vi "Create_Turbulence_Statistics.vi"() -> ()   [LabVIEW 2011]
uses:
  <vilib>/Analysis/1siggen.llb/Ramp Pattern by Samples.vi
  <vilib>/Utility/file.llb/Write To Spreadsheet File (string).vi
  <vilib>/Analysis/baseanly.llb/Quick Scale 1D.vi
  <vilib>/Analysis/NI_AALBase.lvlib
panel:
  in  "Meas Plane":enum16{"XY", "YZ", "XZ"}(ring)
  in  "Invert V":bool
  in  "Invert U":bool
  in  "Output Directory":path=path "C:/Experiments10/NACA0015_D"
  out "Current vector filename":string
  out "v4 (m4/s4)":dbl(graph)
  out "v3 (m3/s3)":dbl(graph)
  out "v2 (m2/s2)":dbl(graph)
  out "V (m/s)":dbl(graph)
  out "v (m/s)":dbl(graph)
  out "u4 (m4/s4)":dbl(graph)
  out "u3 (m3/s3)":dbl(graph)
  out "u2 (m2/s2)":dbl(graph)
  out "u (m/s)":dbl(graph)
  out "U (m/s)":dbl(graph)
  in  "New Filename":string
  in  "Insight 3G File Folder":path=path "C:/Experiments10/NACA0015_D"
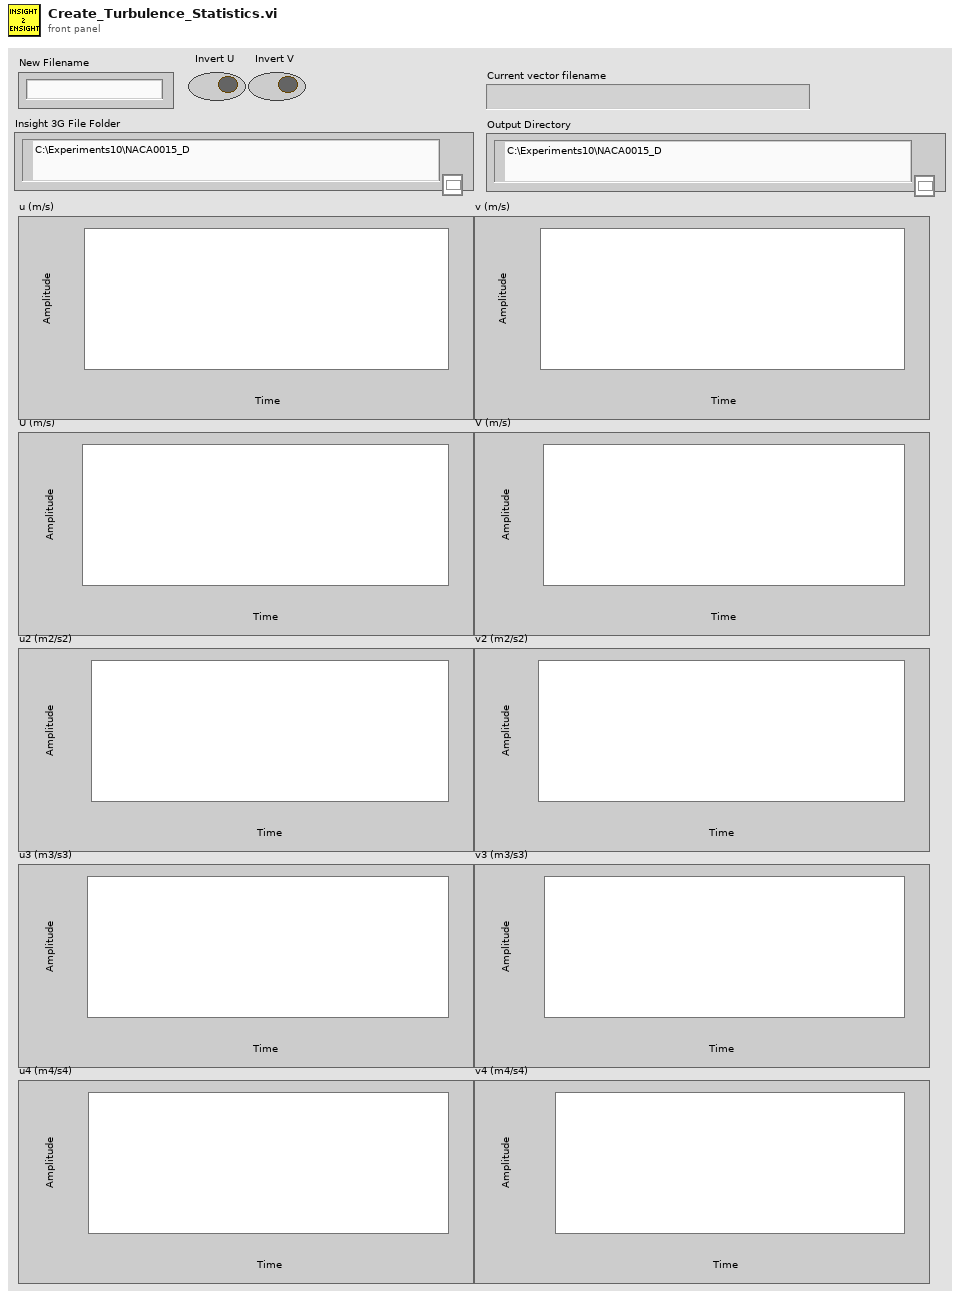
[diagram p1: front panel]
types:
  T1 = cluster{"U m/s":dbl, "u2 m2/s2":dbl, "u3 m3/s3":dbl, "u4 m4/s4":dbl, "TurbU %":dbl, "Skew_u":dbl, "Kurt_u":dbl, "V m/s":dbl, "v2 m2/s2":dbl, "v3 m3/s3":dbl, "v4 m4/s4":dbl, "TurbV %":dbl, "Skew_v":dbl, "Kurt_v":dbl, "u2v2 m4/s4":dbl, "uv3 m4/s4":dbl, "u3v m4/s4":dbl, "uv2 m3/s3":dbl, "u2v m3/s3":dbl, "uv_cc":dbl, "uv":dbl, "TKE J":dbl}
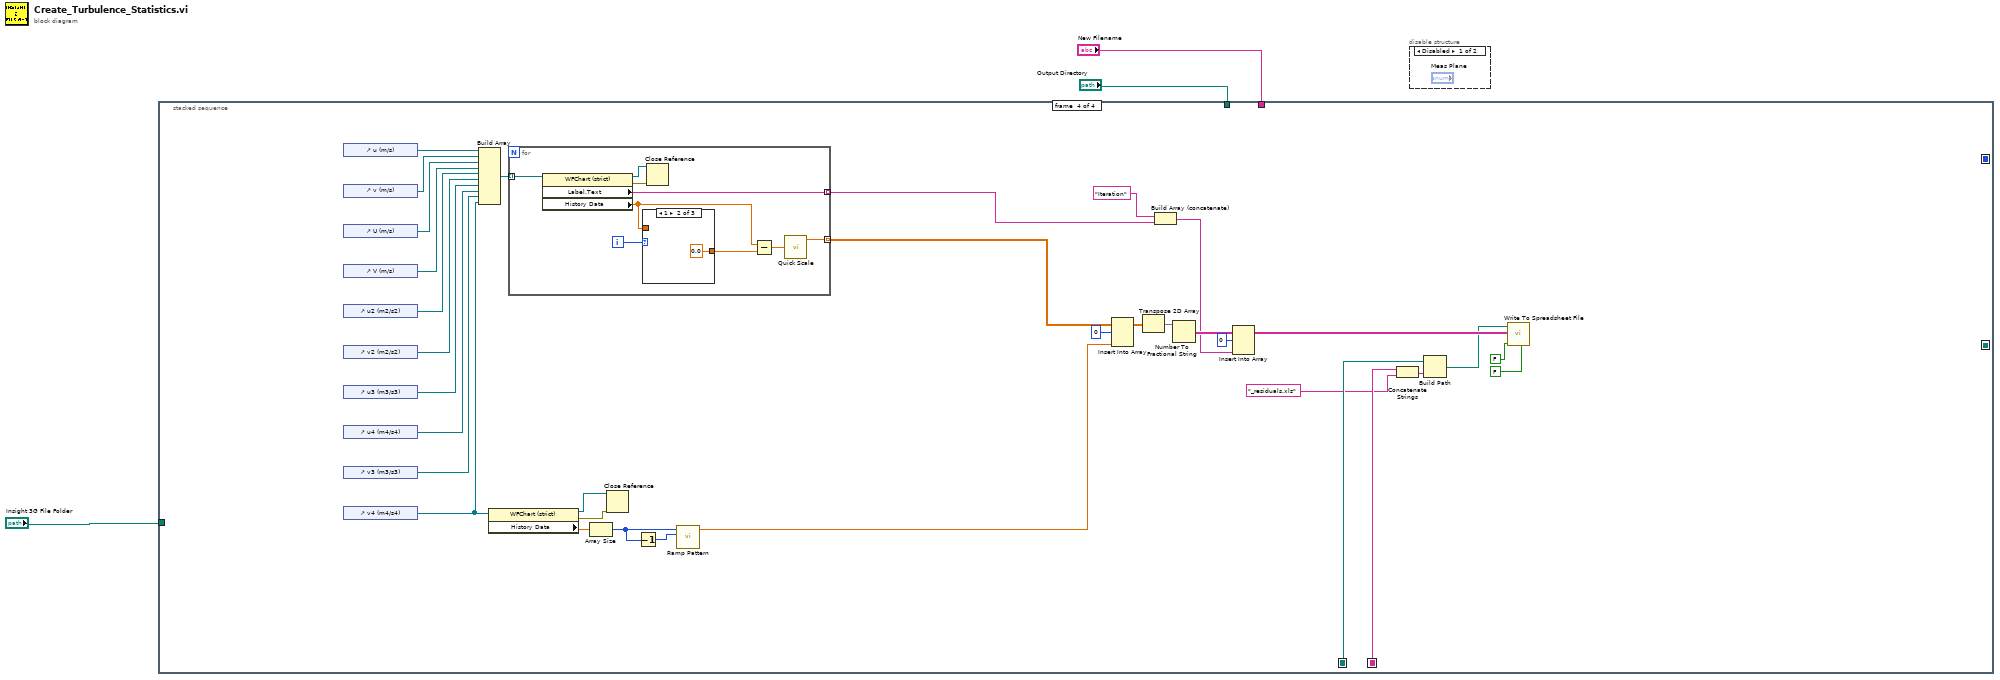
[diagram p0: block diagram]
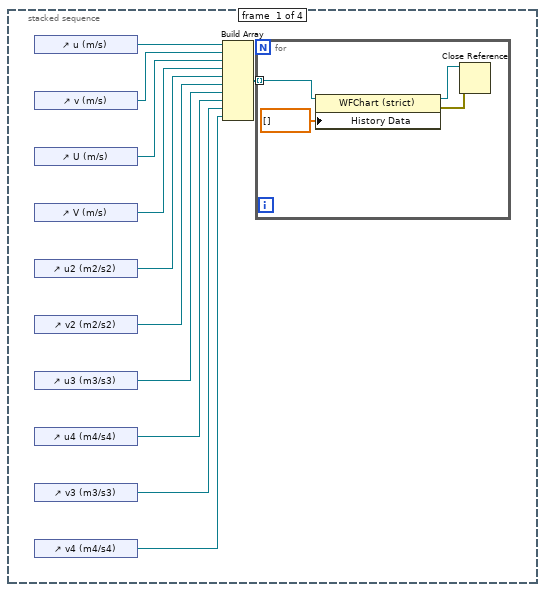
[diagram p3: hidden frame]
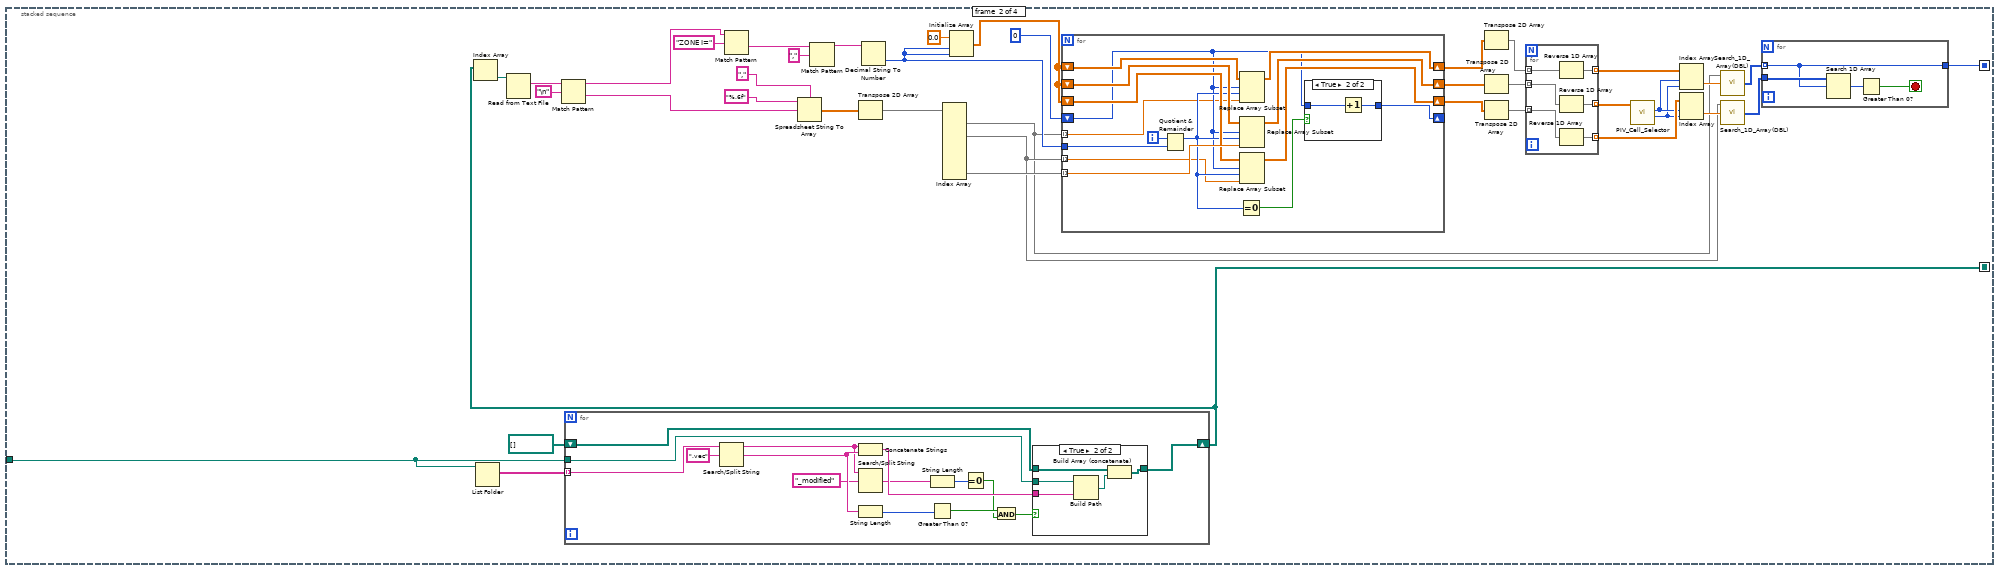
[diagram p4: hidden frame]
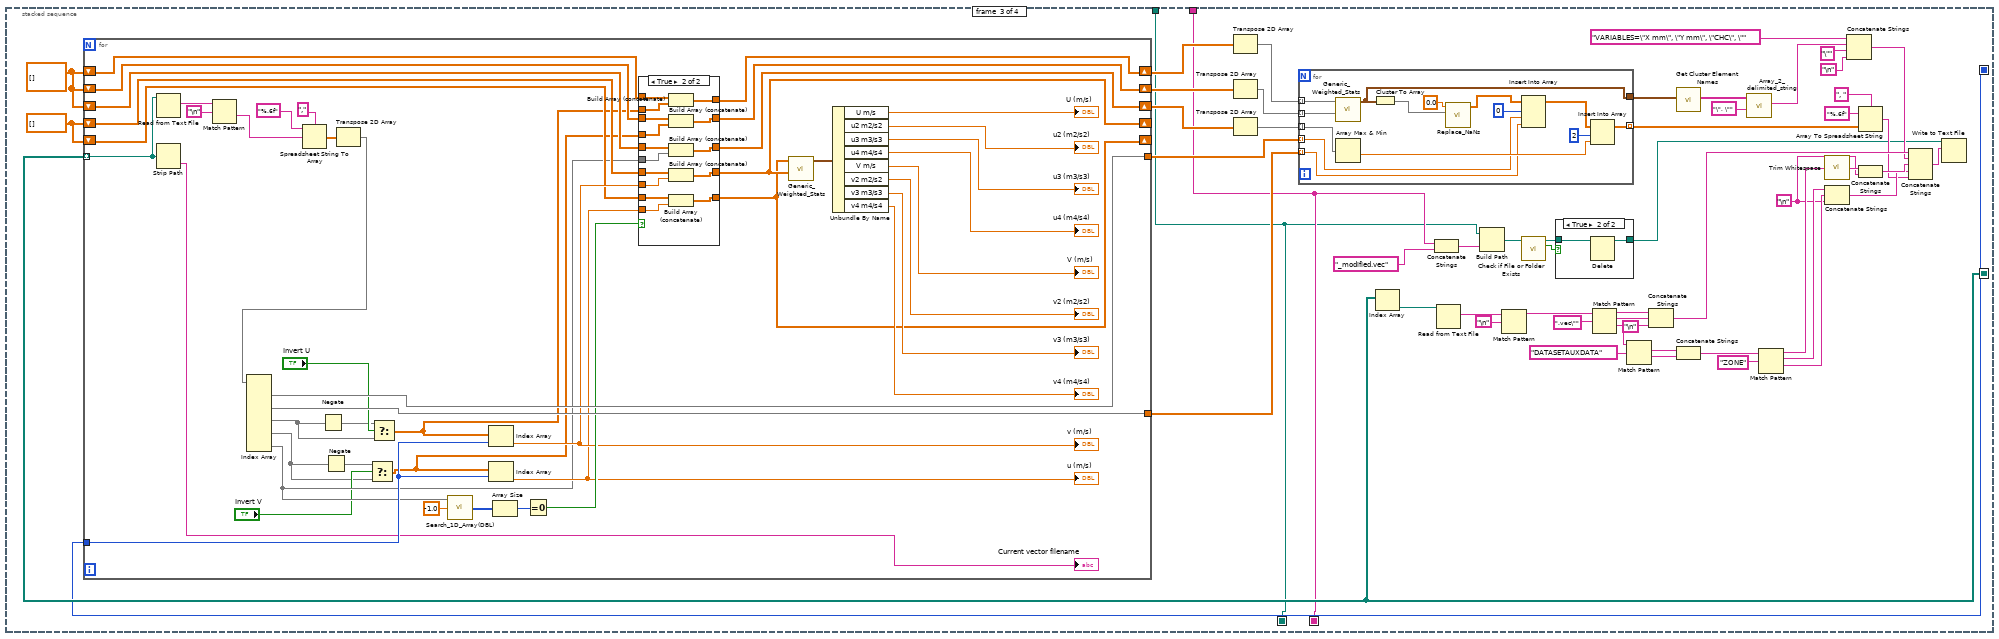
[diagram p7: hidden frame]
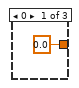
[diagram p10: hidden frame]
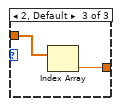
[diagram p11: hidden frame]
diagram:
  n1 = stacked-sequence {
    seq-local: [_ w56 _ _] -> [_ _ w162 _]
    seq-local: [_ w22 _ _] -> [_ _ w161 _]
    seq-local: [_ _ w108 _] -> [_ _ _ w253]
    seq-local: [_ _ w109 _] -> [_ _ _ w249]
    tunnel: "New Filename" -> [_ _ w109 _]
    tunnel: "Output Directory" -> [_ _ w108 _]
    tunnel: "Insight 3G File Folder" -> [_ w19 _ _]
    frame #0 {
      n2 = control-ref of="u (m/s)"() -> (w14:refnum<vi>)
      n3 = control-ref of="v (m/s)"() -> (w13:refnum<vi>)
      n4 = control-ref of="U (m/s)"() -> (w12:refnum<vi>)
      n5 = control-ref of="V (m/s)"() -> (w11:refnum<vi>)
      n6 = control-ref of="u2 (m2/s2)"() -> (w10:refnum<vi>)
      n7 = control-ref of="v2 (m2/s2)"() -> (w9:refnum<vi>)
      n8 = control-ref of="u3 (m3/s3)"() -> (w8:refnum<vi>)
      n9 = control-ref of="u4 (m4/s4)"() -> (w7:refnum<vi>)
      n10 = control-ref of="v3 (m3/s3)"() -> (w6:refnum<vi>)
      n11 = control-ref of="v4 (m4/s4)"() -> (w4:refnum<vi>)
      n12 = Build Array(w14, w13, w12, w11, w10, w9, w8, w7, w6, w4) -> (w5:refnum<vi>[])
      n13 = for {
        tunnel: w5 -> [w18] mode=indexing
        n14 = property class="WFChart (strict)"(reference=w18, "History Data"=dbl[] []) -> (reference out=w16:refnum<vi>, error out=w17:errorcluster)  [unwired: 1 in]
        n15 = Close Reference(reference=w16, error in (no error)=w17) -> ()  [unwired: 1 out]
      }
    }
    frame #1 {
      n16 = List Folder(path=w19) -> (filenames=w57:string[])  [unwired: 3 in, 3 out]
      n17 = for {
        tunnel: w57 -> [w101] mode=indexing
        shift-right: [w94] -> w56
        shift-left: path[] [] -> [w96]
        tunnel: w19 -> [w95]
        n18 = Search/Split String(string=w101, search string/char (-)=".vec") -> (substring before match=w92:string, match + rest of string=w98:string)  [unwired: 1 in, 1 out]
        n19 = Concatenate Strings(w92, w98) -> (w97:string)
        n20 = Search/Split String(string=w92, search string/char (-)="_modified") -> (match + rest of string=w90:string)  [unwired: 1 in, 2 out]
        n21 = String Length(string=w98) -> (length=w99:i32)
        n22 = Greater Than 0?(x=w99) -> (x > 0?=w93:bool)
        n23 = String Length(string=w90) -> (length=w89:i32)
        n24 = Equal To 0?(x=w89) -> (x = 0?=w88:bool)
        n25 = And(x=w93, y=w88) -> (x .and. y?=w87:bool)
        n26 = case shown="True" w87 {
          tunnel: w97 -> [_ w107]
          tunnel: w96 -> [w102 w103]
          tunnel: w95 -> [_ w106]
          tunnel: [w102 w104] -> w94
          frame False {
          }
          frame True {
            n27 = Build Path(base path=w106, name or relative path=w107) -> (appended path=w105:path)
            n28 = Build Array (concatenate)(w103, w105) -> (w104:path[])
          }
        }
      }
      n29 = Index Array(array=w56) -> (element=w55:path)  [unwired: 1 in]
      n30 = Read from Text File(file (use dialog)=w55) -> (text=w48:string)  [unwired: 3 in, 3 out]
      n31 = Match Pattern(string=w48, regular expression="\n") -> (before substring=w47:string, after substring=w51:string)  [unwired: 1 in, 2 out]
      n32 = Match Pattern(string=w47, regular expression="ZONE I=") -> (after substring=w45:string)  [unwired: 1 in, 3 out]
      n33 = Spreadsheet String To Array(delimiter (Tab)=",", format string="%.6f", spreadsheet string=w51) -> (array=w50:dbl[][])  [unwired: 1 in]
      n34 = Match Pattern(string=w45, regular expression=",") -> (before substring=w43:string)  [unwired: 1 in, 3 out]
      n35 = Transpose 2D Array(2D array=w50) -> (transposed array=w53:dbl[][])
      n36 = Decimal String To Number(string=w43) -> (number=w27:i32)  [unwired: 2 in, 1 out]
      n37 = Index Array(array=w53) -> (element #1=w23:dbl[], element #2=w24:dbl[], element #5=w42:dbl[])  [unwired: 10 in, 2 out]
      n38 = Initialize Array(0.0 ("element"), w27, w27) -> (w36:dbl[][])
      n39 = for {
        tunnel: w42 -> [w79] mode=indexing
        tunnel: w27 -> [w82]
        shift-right: [w80] -> w39
        shift-left: w36 -> [w81]
        shift-right: [w78] -> _
        shift-left: 0 -> [w71]
        shift-right: [w76] -> w34
        shift-left: w36 -> [w75]
        shift-right: [w73] -> w35
        shift-left: w36 -> [w74]
        tunnel: w23 -> [w70] mode=indexing
        tunnel: w24 -> [w69] mode=indexing
        i -> [w83]
        n40 = Quotient & Remainder(x=w83, y=w82) -> (x-y*floor(x/y)=w72:i32)  [unwired: 1 out]
        n41 = Equal To 0?(x=w72) -> (x = 0?=w77:bool)
        n42 = Replace Array Subset(array=w74, new element=w70, index (row)=w71, index (col)=w72) -> (w73:dbl[][])
        n43 = Replace Array Subset(array=w81, new element=w79, index (row)=w71, index (col)=w72) -> (w80:dbl[][])
        n44 = Replace Array Subset(array=w75, new element=w69, index (row)=w71, index (col)=w72) -> (w76:dbl[][])
        n45 = case shown="True" w77 {
          tunnel: [w84 w85] -> w78
          tunnel: w71 -> [w84 w86]
          frame False {
          }
          frame True {
            n46 = Increment(x=w86) -> (x+1=w85:i32)
          }
        }
      }
      n47 = Transpose 2D Array(2D array=w35) -> (transposed array=w33:dbl[][])
      n48 = Transpose 2D Array(2D array=w39) -> (transposed array=w38:dbl[][])
      n49 = Transpose 2D Array(2D array=w34) -> (transposed array=w32:dbl[][])
      n50 = for {
        tunnel: w38 -> [w68] mode=indexing
        tunnel: [w67] -> w37 mode=indexing
        tunnel: w33 -> [w66] mode=indexing
        tunnel: w32 -> [w65] mode=indexing
        tunnel: [w64] -> w30 mode=indexing
        tunnel: [w63] -> w31 mode=indexing
        n51 = Reverse 1D Array(array=w66) -> (reversed array=w63:dbl[])
        n52 = Reverse 1D Array(array=w68) -> (reversed array=w67:dbl[])
        n53 = Reverse 1D Array(array=w65) -> (reversed array=w64:dbl[])
      }
      n54 = call "PIV_Cell_Selector.vi"("CHC"=w37) -> ("Y Index"=w20:i32, "X Index"=w21:i32)  [unwired: 9 in]
      n55 = Index Array(array=w31, index (row)=w21, index (col)=w20) -> (element=w29:dbl)
      n56 = Index Array(array=w30, index (row)=w21, index (col)=w20) -> (element=w28:dbl)
      n57 = call "Search_1D_Array(DBL).vi"("Array"=w23, "Element Data"=w29) -> ("Indicies of Elements"=w26:i32[])  [unwired: 7 in]
      n58 = call "Search_1D_Array(DBL).vi"("Array"=w24, "Element Data"=w28) -> ("Indicies of Elements"=w25:i32[])  [unwired: 7 in]
      n59 = for {
        tunnel: w26 -> [w59] mode=indexing
        tunnel: w25 -> [w62]
        tunnel: [w59] -> w22
        stop <- w60 stop-if-true
        n60 = Search 1D Array(1D array=w62, element=w59) -> (index of element=w61:i32)  [unwired: 1 in]
        n61 = Greater Than 0?(x=w61) -> (x > 0?=w60:bool)
      }
    }
    frame #2 {
      w114 = dbl[][] []
      w115 = dbl[] []
      w134 = "\n"
      n62 = for {
        tunnel: w162 -> [w204] mode=indexing
        tunnel: [w218] -> w123
        tunnel: [w217] -> w122
        tunnel: w161 -> [w216]
        shift-right: [w194] -> _
        shift-left: w115 -> [w195]
        shift-right: [w197] -> _
        shift-left: w115 -> [w198]
        shift-right: [w189] -> w112
        shift-left: w114 -> [w191]
        shift-right: [w188] -> w111
        shift-left: w114 -> [w190]
        shift-right: [w193] -> w113
        shift-left: w114 -> [w200]
        n63 = Read from Text File(file (use dialog)=w204) -> (text=w221:string)  [unwired: 3 in, 3 out]
        n64 = Strip Path(path=w204) -> (name=→"Current vector filename":string)  [unwired: 1 out]
        n65 = Match Pattern(string=w221, regular expression="\n") -> (after substring=w220:string)  [unwired: 1 in, 3 out]
        n66 = Spreadsheet String To Array(delimiter (Tab)=",", format string="%.6f", spreadsheet string=w220) -> (array=w219:dbl[][])  [unwired: 1 in]
        n67 = Transpose 2D Array(2D array=w219) -> (transposed array=w223:dbl[][])
        n68 = Index Array(array=w223) -> (element #1=w218:dbl[], element #2=w217:dbl[], element #3=w185:dbl[], element #4=w181:dbl[], element #5=w192:dbl[])  [unwired: 10 in]
        n69 = Negate(x=w185) -> (-x=w184:dbl[])
        n70 = Negate(x=w181) -> (-x=w180:dbl[])
        n71 = Select(t=w180, s="Invert V", f=w181) -> (s? t:f=w183:dbl[])
        n72 = Select(t=w184, s="Invert U", f=w185) -> (s? t:f=w186:dbl[])
        n73 = call "Search_1D_Array(DBL).vi"("Array"=w192, "Element Data"=-1.0) -> ("Indicies of Elements"=w205:i32[])  [unwired: 7 in]
        n74 = Index Array(array=w186, index=w216) -> (element=w199:dbl)
        "v (m/s)" <- w199
        n75 = Index Array(array=w183, index=w216) -> (element=w196:dbl)
        "u (m/s)" <- w196
        n76 = Array Size(array=w205) -> (size(s)=w202:i32)
        n77 = Equal To 0?(x=w202) -> (x = 0?=w201:bool)
        n78 = case shown="True" w201 {
          tunnel: w200 -> [w228 w238]
          tunnel: w199 -> [_ w245]
          tunnel: w198 -> [w229 w244]
          tunnel: [w229 w243] -> w197
          tunnel: w196 -> [_ w242]
          tunnel: w195 -> [w230 w241]
          tunnel: [w230 w240] -> w194
          tunnel: w186 -> [_ w239]
          tunnel: [w228 w237] -> w193
          tunnel: w183 -> [_ w236]
          tunnel: w192 -> [_ w235]
          tunnel: w191 -> [w227 w234]
          tunnel: w190 -> [w226 w233]
          tunnel: [w227 w232] -> w189
          tunnel: [w226 w231] -> w188
          frame False {
          }
          frame True {
            n79 = Build Array (concatenate)(w238, w239) -> (w237:dbl[][])
            n80 = Build Array (concatenate)(w234, w236) -> (w232:dbl[][])
            n81 = Build Array (concatenate)(w233, w235) -> (w231:dbl[][])
            n82 = Build Array (concatenate)(w244, w245) -> (w243:dbl[])
            n83 = Build Array (concatenate)(w241, w242) -> (w240:dbl[])
          }
        }
        n84 = call "Generic_Weighted_Stats.vi"("v"=w197, "u"=w194) -> ("Turbulence Statistics"=w215:T1)  [unwired: 9 in]
        n85 = Unbundle By Name(w215) -> ("U m/s"=→"U (m/s)":dbl, "u2 m2/s2"=→"u2 (m2/s2)":dbl, "u3 m3/s3"=→"u3 (m3/s3)":dbl, "u4 m4/s4"=→"u4 (m4/s4)":dbl, "V m/s"=→"V (m/s)":dbl, "v2 m2/s2"=→"v2 (m2/s2)":dbl, "v3 m3/s3"=→"v3 (m3/s3)":dbl, "v4 m4/s4"=→"v4 (m4/s4)":dbl)
      }
      n86 = Transpose 2D Array(2D array=w113) -> (transposed array=w160:dbl[][])
      n87 = Transpose 2D Array(2D array=w112) -> (transposed array=w159:dbl[][])
      n88 = Transpose 2D Array(2D array=w111) -> (transposed array=w124:dbl[][])
      n89 = for {
        tunnel: w160 -> [w179] mode=indexing
        tunnel: w159 -> [w178] mode=indexing
        tunnel: [w174] -> w128 mode=indexing
        tunnel: w123 -> [w172] mode=indexing
        tunnel: w122 -> [w173] mode=indexing
        tunnel: w124 -> [w176] mode=indexing
        tunnel: [w166] -> w117
        n90 = call "Generic_Weighted_Stats.vi"("v"=w178, "u"=w179) -> ("Turbulence Statistics"=w166:T1)  [unwired: 9 in]
        n91 = Array Max & Min(array=w176) -> (min value=w175:dbl)  [unwired: 3 out]
        n92 = Cluster To Array(cluster=w166) -> (array=w169:dbl[])
        n93 = call "Replace_NaNs.vi"("Array"=w169, "Replacement"=0.0 ("t")) -> ("Array Out"=w168:dbl[])  [unwired: 9 in]
        n94 = Insert Into Array(array=w168, index=0, new element #1=w172, new element #2=w173) -> (w170:dbl[])
        n95 = Insert Into Array(array=w170, index=2, new element=w175) -> (w174:dbl[])
      }
      n96 = Index Array(array=w162) -> (element=w154:path)  [unwired: 1 in]
      n97 = Concatenate Strings(w109, "_modified.vec" ("string")) -> (w110:string)
      n98 = Read from Text File(file (use dialog)=w154) -> (text=w157:string)  [unwired: 3 in, 3 out]
      n99 = Build Path(base path=w108, name or relative path=w110) -> (appended path=w133:path)
      n100 = Match Pattern(string=w157, regular expression="\n") -> (before substring=w156:string)  [unwired: 1 in, 3 out]
      n101 = call <vilib>:"Check if File or Folder Exists.vi"("path"=w133) -> ("file or folder exists?"=w120:bool, "dup path"=w119:path)  [unwired: 8 in, 1 out]
      n102 = case shown="True" w120 {
        tunnel: w119 -> [w163 w165]
        tunnel: [w163 w164] -> w118
        frame False {
        }
        frame True {
          n103 = Delete(path (use dialog)=w165) -> (deleted path=w164:path)  [unwired: 4 in, 2 out]
        }
      }
      n104 = Match Pattern(string=w156, regular expression=".vec\"") -> (before substring=w151:string, match substring=w150:string, after substring=w148:string)  [unwired: 1 in, 1 out]
      n105 = Match Pattern(string=w148, regular expression="DATASETAUXDATA") -> (match substring=w146:string, after substring=w145:string)  [unwired: 1 in, 2 out]
      n106 = Concatenate Strings(w151, w150, "\n") -> (w138:string)
      n107 = call "Get Cluster Element Names.vi"("Cluster"=w117) -> ("Element Names"=w116:string[])  [unwired: 9 in, 1 out]
      n108 = Concatenate Strings(w146, w145) -> (w144:string)
      n109 = call "Array_2_delimited_string.vi"("delimiter (Tab)"="\", \"", "Array of Strings"=w116) -> ("delimited string"=w131:string)  [unwired: 9 in]
      n110 = Match Pattern(string=w144, regular expression="ZONE") -> (before substring=w142:string, match substring=w140:string, after substring=w139:string)  [unwired: 1 in, 1 out]
      n111 = call <vilib>:"Trim Whitespace.vi"("string"=w142) -> ("trimmed string"=w141:string)  [unwired: 1 in]
      n112 = Concatenate Strings(w140, w139, w134) -> (w135:string)
      n113 = Concatenate Strings("VARIABLES=\"X mm\", \"Y mm\", \"CHC\", \"" ("string"), w131, "\"" ("string"), "\n") -> (w137:string)
      n114 = Array To Spreadsheet String(delimiter (Tab)=", ", array=w128, 3:"%.6f" ("format string")) -> (spreadsheet string=w125:string)
      n115 = Concatenate Strings(w141, w134) -> (w136:string)
      n116 = Concatenate Strings(w138, w137, w136, w135, w125) -> (w121:string)
      n117 = Write to Text File(file (use dialog)=w118, text=w121) -> ()  [unwired: 2 in, 3 out]
    }
    frame #3 {
      n118 = control-ref of="u (m/s)"() -> (w279:refnum<vi>)
      n119 = control-ref of="v (m/s)"() -> (w278:refnum<vi>)
      n120 = control-ref of="U (m/s)"() -> (w277:refnum<vi>)
      n121 = control-ref of="V (m/s)"() -> (w276:refnum<vi>)
      n122 = control-ref of="u2 (m2/s2)"() -> (w275:refnum<vi>)
      n123 = control-ref of="v2 (m2/s2)"() -> (w274:refnum<vi>)
      n124 = control-ref of="u3 (m3/s3)"() -> (w273:refnum<vi>)
      n125 = control-ref of="u4 (m4/s4)"() -> (w272:refnum<vi>)
      n126 = control-ref of="v3 (m3/s3)"() -> (w271:refnum<vi>)
      n127 = control-ref of="v4 (m4/s4)"() -> (w269:refnum<vi>)
      n128 = Build Array(w279, w278, w277, w276, w275, w274, w273, w272, w271, w269) -> (w270:refnum<vi>[])
      n129 = property class="WFChart (strict)"(reference=w269) -> (reference out=w267:refnum<vi>, error out=w266:errorcluster, "History Data"=w268:dbl[])  [unwired: 1 in]
      n130 = for {
        tunnel: w270 -> [w288] mode=indexing
        tunnel: [w281] -> w264 mode=indexing
        tunnel: [w287] -> w260 mode=indexing
        i -> [w280]
        n131 = property class="WFChart (strict)"(reference=w288) -> (reference out=w285:refnum<vi>, error out=w286:errorcluster, "Label.Text"=w287:string, "History Data"=w284:dbl[])  [unwired: 1 in]
        n132 = case shown="1" w280 {
          tunnel: w284 -> [_ _ w292]
          tunnel: [0.0 0.0 w291] -> w283
          frame 0 {
          }
          frame 1 {
          }
          frame 2, Default {
            n133 = Index Array(array=w292) -> (element=w291:dbl)  [unwired: 1 in]
          }
        }
        n134 = Close Reference(reference=w285, error in (no error)=w286) -> ()  [unwired: 1 out]
        n135 = Subtract(x=w284, y=w283) -> (x-y=w282:dbl[])
        n136 = call-poly <vilib>:"Quick Scale.vi"("X"=w282) -> ("Y[i]=X[i]/Max|X|"=w281:dbl[])  [unwired: 2 out]
      }
      n137 = Array Size(array=w268) -> (size(s)=w265:i32)
      n138 = Close Reference(reference=w267, error in (no error)=w266) -> ()  [unwired: 1 out]
      n139 = Decrement(x=w265) -> (x-1=w246:i32)
      n140 = call-poly <vilib>:"Ramp Pattern.vi"("end"=w246, "samples"=w265) -> ("Ramp Pattern"=w263:dbl[])  [unwired: 8 in, 1 out]
      n141 = Insert Into Array(array=w264, index (row)=0, new element=w263) -> (w261:dbl[][])  [unwired: 1 in]
      n142 = Transpose 2D Array(2D array=w261) -> (transposed array=w258:dbl[][])
      n143 = Build Array (concatenate)("Iteration", w260) -> (w256:string[])
      n144 = Number To Fractional String(number=w258) -> (F-format string=w257:string[][])  [unwired: 3 in]
      n145 = Insert Into Array(array=w257, index (row)=0, new element=w256) -> (w254:string[][])  [unwired: 1 in]
      n146 = Concatenate Strings(w249, "_residuals.xls" ("string")) -> (w248:string)
      n147 = Build Path(base path=w253, name or relative path=w248) -> (appended path=w252:path)
      n148 = call-poly <vilib>:"Write To Spreadsheet File.vi"("transpose? (no:F)"=FALSE, "append to file? (new file:F)"=FALSE, "2D data"=w254, "file path (dialog if empty)"=w252) -> ()  [unwired: 4 in, 1 out]
    }
  }
  n149 = disable-structure shown="Disabled" {
    frame Disabled {
    }
    frame Enabled {
    }
  }
